vi "Simple Motor Test.vi"   [LabVIEW 2009]
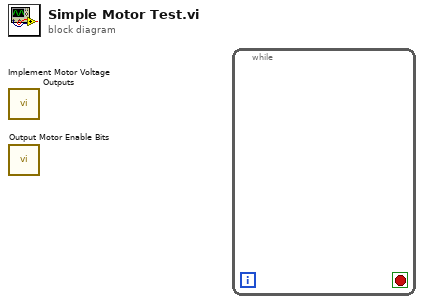
[diagram p0: block diagram]
diagram:
  n1 = call "Implement Motor Voltage Outputs.vi"() -> ()  [unwired: 1 in]
  n2 = call "Output Motor Enable Bits.vi"() -> ()  [unwired: 1 in]
  n3 = while {
    stop <- _ stop-if-true
  }
